vi "SRCleaner(SubVI).vi"(8 "error in (no error)":errorcluster, 11 "Data Value Reference in":refnum<data-value>) -> (0 "error out":errorcluster, 3 "Data Value Reference out":refnum<data-value>)   [LabVIEW 2016]
uses:
  Modules/Private Controls/Report Data Cluster.ctl
  Modules/Private Controls/Data Raw.ctl
  Modules/Data Operations.lvlib
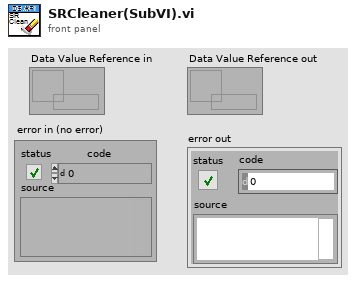
[diagram p1: front panel]
types:
  T1 = typedef "Data Operations.lvlib/Report Data Cluster.ctl" = cluster{"Headers":cluster{"Start Date":timestamp, "End Date":timestamp, "SR Status String":string[], "AE Owner String":string[]}, "Data":T2[]}
  T2 = typedef "Data Operations.lvlib/Data Raw.ctl" = cluster{"SR Number":string, "Status":string, "Summary":string, "AE Owner":string, "AE Group":string, "Contact":string, "SurveyData":cluster{"Resolution Time":dbl, "Total Satisfaction":dbl, "Response Time":dbl, "Courtesy":dbl, "Problem Solved":dbl}, "Time Data":cluster{"Last Update Date":timestamp, "Request Date":timestamp, "Request week":u8}}
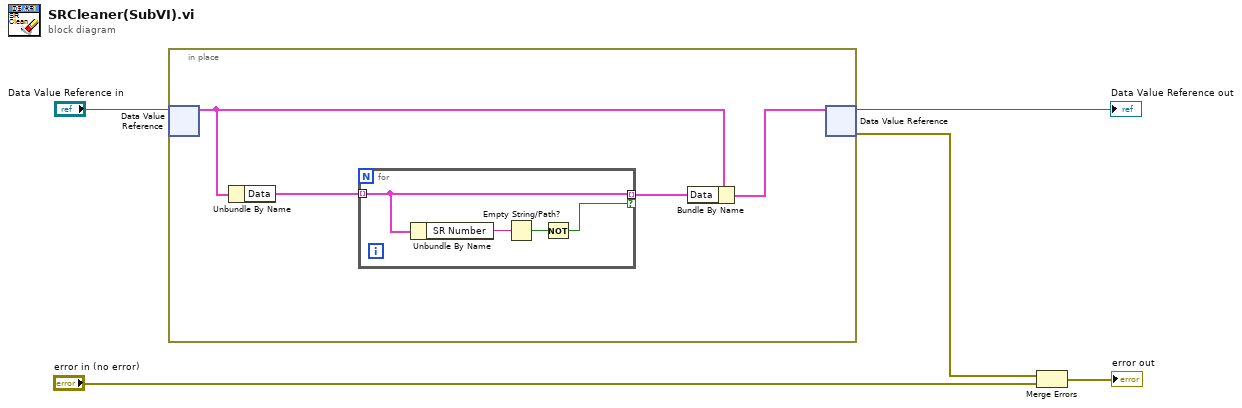
[diagram p0: block diagram]
diagram:
  n1 = in-place {
    n2 = in-place-dvr #1("Data Value Reference in") -> (w8:T1)  [unwired: 1 out]
    n3 = Unbundle By Name(w8) -> ("Data"=w9:T2[])
    n4 = for {
      tunnel: w9 -> [w12] mode=indexing
      tunnel: [w12] -> w6 mode=indexing if=w10
      n5 = Unbundle By Name(w12) -> ("SR Number"=w13:string)
      n6 = Empty String/Path?(string/path=w13) -> (empty?=w11:bool)
      n7 = Not(x=w11) -> (.not. x?=w10:bool)
    }
    n8 = Bundle By Name(cluster=w8, "Data"=w6) -> (w7:T1)
    n9 = in-place-dvr #1(w7) -> (→"Data Value Reference out":refnum<data-value>, w2:errorcluster)
  }
  n10 = Merge Errors(w2, "error in (no error)") -> (→"error out":errorcluster)
